vi "setParameters.vi"(10 "Parameters":T1, 11 "ExitCommand in":refnum<class "ExitCommand.lvclass">) -> (3 "ExitCommand out":refnum<class "ExitCommand.lvclass">)   [LabVIEW 2016, in "ExitCommand.lvclass"]
uses:
  ExitCommand.lvclass
  Communicator/Topics/CommandExit.ctl
  Communicator/Topics/CommandId.ctl
  ExitCommand.lvclass/ExitCommand.ctl
  Communicator/M1M3Communicator.lvlib
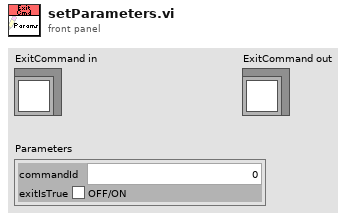
[diagram p1: front panel]
types:
  T1 = typedef "M1M3Communicator.lvlib/CommandExit.ctl" = cluster{"commandId":T2, "exitIsTrue":bool}
  T2 = typedef "M1M3Communicator.lvlib/CommandId.ctl" = i32
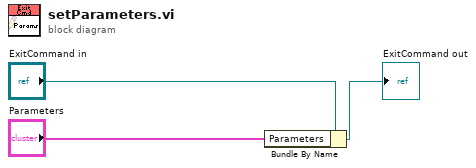
[diagram p0: block diagram]
diagram:
  n1 = Bundle By Name(cluster="ExitCommand in", "Parameters"="Parameters") -> (→"ExitCommand out":refnum<class "ExitCommand.lvclass">)
